vi "FPGA VI_16 Channels_High Speed.vi"() -> ()   [LabVIEW 2015]
uses:
  Types/Injector.Timing.ctl
  Types/Injection.Core.Settings.ctl
  Types/Injection.Global.Settings.ctl
  <vilib>/rvi/eio/common/nirviEmuClasses.ctl
  <vilib>/Platform/TimedLoop/XDataNode/timing_clust.ctl
  <vilib>/Platform/TimedLoop/XDataNode/nitl_modes.ctl
  <vilib>/Platform/TimedLoop/XDataNode/wakeup.ctl
  Types/Injection.Core.Internal.Settings.ctl
  <vilib>/rvi/eio/common/nirviEmuTemplateMethod_errors.vi
  <vilib>/rvi/Emulation/niFpgaGetClockAttributes.vi
  <vilib>/rvi/Emulation/niFpgaSctlEmulationGetInTimedLoop.vi
  <vilib>/rvi/Emulation/niFpgaEmulationReportErrorSimple.vi
  <vilib>/rvi/Emulation/niFpgaCriticalErrorInLSC.vi
  <vilib>/rvi/eio/common/nirviEmuTemplateMethod_noerrors.vi
  <vilib>/rvi/DataTransferAndStorage/Container/Common/niFpgaContainerExecOnDevCompGetState.vi
  <vilib>/rvi/Emulation/niFpgaEmulationIsFPGAContextNoSignature.vi
  <vilib>/rvi/errors/niFpgaSetErrorForExecOnDevCompSimple.vi
  <vilib>/rvi/eio/common/nirviEmuReportErrorAndStop.vi
  <vilib>/rvi/DataTransferAndStorage/Container/Common/niFpgaContainerGetUniqueNameForEmu.vi
  <vilib>/rvi/FIFO/Fifo_Resource/nirvififoEmulationSetSize.vi
  <vilib>/rvi/FIFO/Fifo_Resource/nirviFifoEmulationQueueMgr.vi
  <instcachedir>/0/nirviFifoEmulationQueueMgr_E5CAEC123FF24DC58D834DCA3CDAA9B5.lvgen/nirviFifoEmulationQueueMgr_E5CAEC123FF24DC58D834DCA3CDAA9B5_010.vi
  <vilib>/rvi/FIFO/Fifo_Resource/nirvififoEmulationDetermineInputValidOut.vi
  <vilib>/rvi/FIFO/Fifo_Resource/nirvififoEmulationCreateLock.vi
  <vilib>/rvi/Emulation/niFpgaProcessEmulError.vi
  <vilib>/rvi/FIFO/Fifo_Resource/nirvififoEmulationObtainLock.vi
  <vilib>/rvi/FIFO/Fifo_Resource/nirvififoEmulationReleaseLock.vi
  <vilib>/rvi/occurrence/nirviWaitOnOccurrenceBase.vi
  <vilib>/rvi/errors/nirviReportUnexpectedCaseInternalError.vi
  <vilib>/rvi/errors/nirviReportUnexpectedCaseInternalError (U32).vi
  <vilib>/Utility/error.llb/Clear Errors.vi
  <vilib>/rvi/interface/RandomDataEmulation/niFpgaRandomDataHandleErrors.vi
  <instcachedir>/0/nirviFifoEmulationQueueMgr_E5CAEC123FF24DC58D834DCA3CDAA9B5.lvgen/nirviFifoEmulationQueueMgr_E5CAEC123FF24DC58D834DCA3CDAA9B5_008.vi
  <vilib>/eio/EIOGrowableMethodNode/genericMethod/EIOGrowableMethodNode.xnode
  <vilib>/rvi/eio/nirviEIOMethodImplementation/nirviEIOMethodImplementation.xnode
  <vilib>/rvi/eio/nirviErrorMerge/nirviErrorMerge.xnode
  <vilib>/Platform/TimedLoop/XDataNode/XDataNode.xnode
  <vilib>/rvi/DataTransferAndStorage/Container/XNode/niFpgaContainer.xnode
  <vilib>/rvi/FIFO/Fifo_Resource/niFpgaFifoEmulationRefIn.vi
  <vilib>/rvi/interface/RandomDataEmulation/nirviRandomDataFpgaReadWriteTemplate.vi
  <vilib>/Platform/TimedLoop/XDataNode/XDNodeRunTimeDep.lvlib
panel:
  out "Sample Clock Ticks":u32
  out "Module Error":bool
  out "Module Initialization Error Code":i32
  out "IO Node Timeout":bool
  in  "Settings.Index12.Injector12":T1
  in  "Settings.Index13.Injector13":T1
  in  "Settings.Index14.Injector14":T1
  in  "Settings.Index15.Injector15":T1
  in  "Settings.Index6.Injector6":T1
  in  "Settings.Index7.Injector7":T1
  in  "Settings.Index8.Injector8":T1
  in  "Settings.Index9.Injector9":T1
  in  "Settings.Index10.Injector10":T1
  in  "Settings.Index11.Injector11":T1
  out "Intermediate FIFO Write Timeout":bool
  in  "Settings.Global":T2={"Enable?"=FALSE, "Initial Voltage Threshold"=12.0, "Event Dwell Limit"=2000, "Voltage Gain"=1.0, "Current Gain"=1.0}
  in  "Settings.Index0.Injector0":T1
  in  "Settings.Index1.Injector1":T1
  in  "Settings.Index2.Injector2":T1
  in  "Settings.Index3.Injector3":T1
  in  "Settings.Index4.Injector4":T1
  in  "Settings.Index5.Injector5":T1
  in  "Settings.Timing":T3={"Injector Sample Period (Ticks)"=80}
  out "Acqusition Loop Ticks":u32
  in  "Settings.DMA":cluster{"# of Injectors":u8}={"# of Injectors"=16}
  out "Host DMA Out?":bool
  out "Intermediate Time Out?":bool
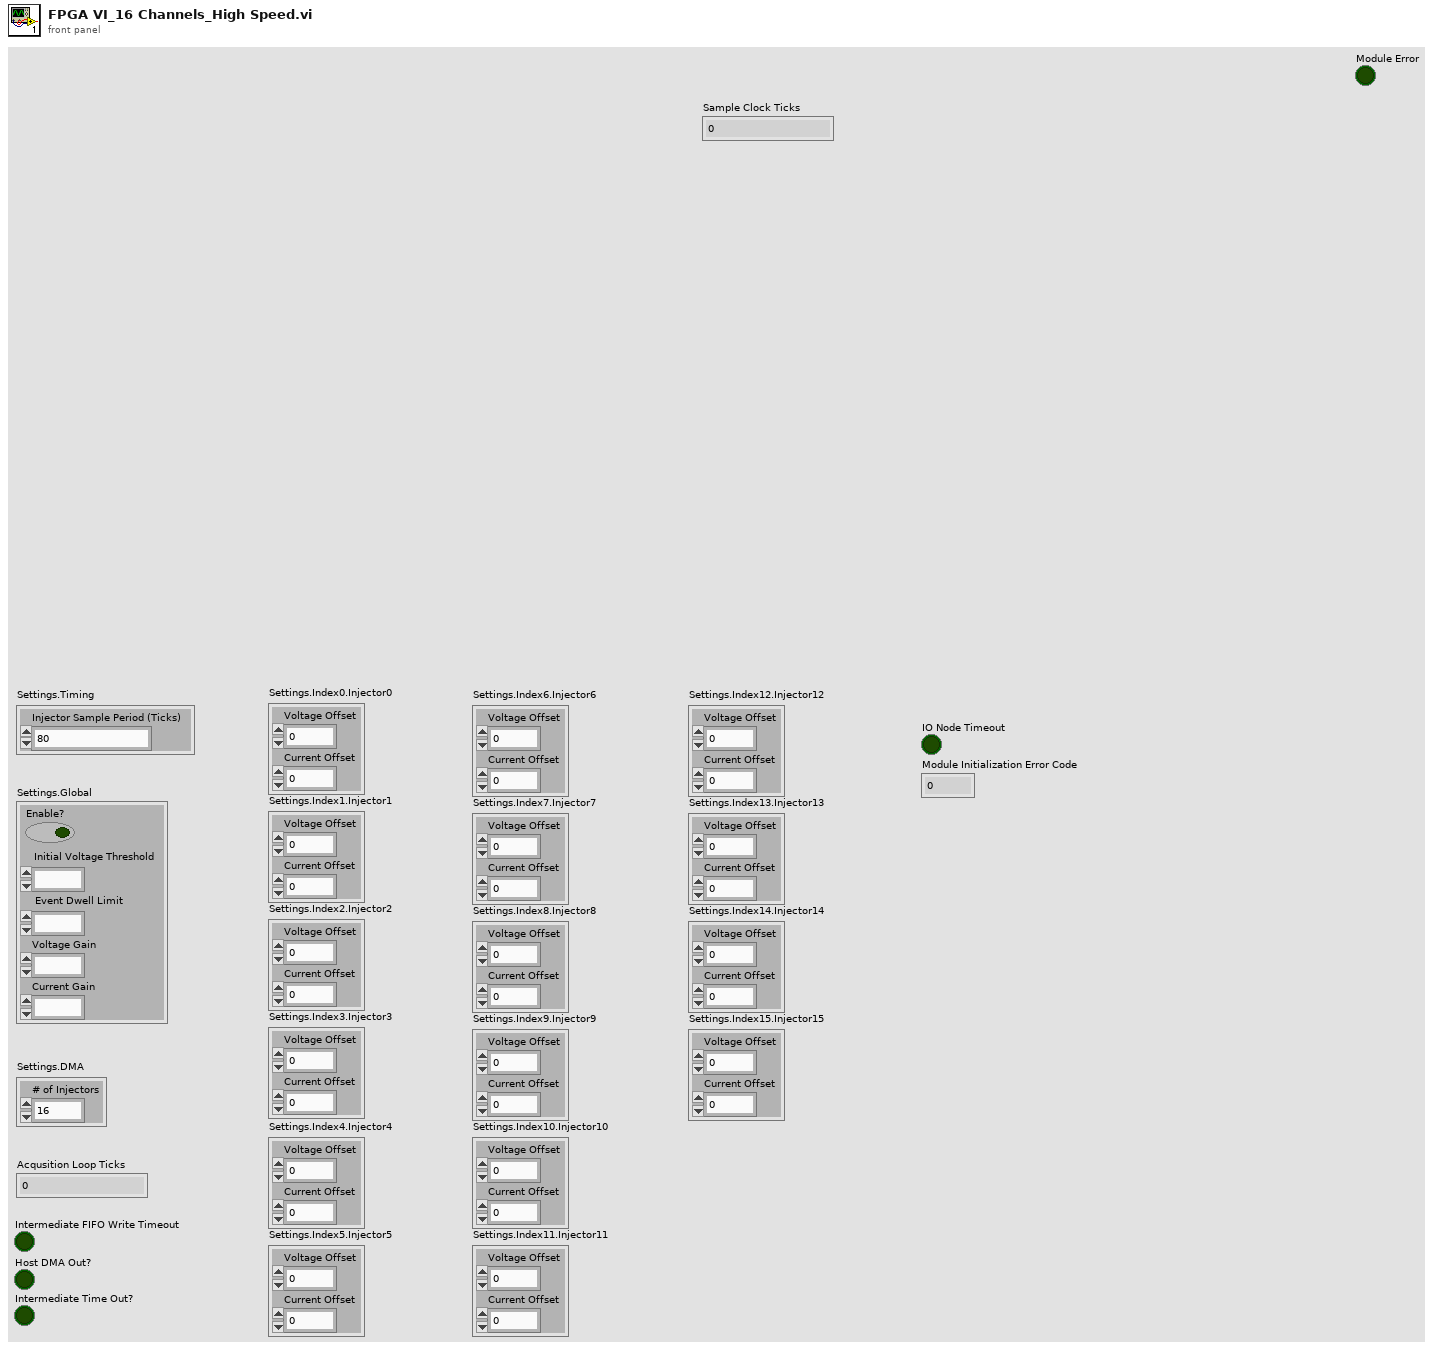
[diagram p1: front panel]
types:
  T1 = typedef "Injection.Core.Settings.ctl" = cluster{"Voltage Offset":fxp<+/-,32,8>, "Current Offset":fxp<+/-,32,8>}
  T2 = typedef "Injection.Global.Settings.ctl" = cluster{"Enable?":bool, "Initial Voltage Threshold":fxp<+/-,32,8>, "Event Dwell Limit":u16, "Voltage Gain":fxp<+/-,32,8>, "Current Gain":fxp<+/-,32,8>}
  T3 = typedef "Injector.Timing.ctl" = cluster{"Injector Sample Period (Ticks)":u32}
  T4 = typedef "nirviEmuClasses.ctl" = enum16{"IO Read", "IO Write", "Method", "Property Read", "Property Write"}
  T5 = cluster{"Data.Samples":u32, "Injection.Period":u32, "Injector.Index":u8, "Iteration":u32}
  T6 = enum8{"Wait on Transfer", "Transfer Injector Index", "Transfer # of Samples", "Transfer Injection Period", "Transfer Data Samples"}
  T7 = typedef "XDNodeRunTimeDep.lvlib/timing_clust.ctl" = cluster{"Expected End [f-1]":u64, "Actual End [f-1]":u64, "Finished Late? [f-1]":bool, "Expected End [i-1]":u64, "Actual End [i-1]":u64, "Finished Late? [i-1]":bool, "Expected Start [i]":u64, "Actual Start [i]":u64, "Expected Start [f]":u64, "Actual Start [f]":u64, "Source Name":string, "Structure Name":string, "Period":i64, "Deadline":i64, "Offset":i64, "Start":i64, "Priority":i32, "Timeout":i32, "Mode":T8, "Wakeup Reason":T9, "Error":errorcluster, "Source Type":string, "Secondary Source Type":string, "Global End Time":u64, "Global Start Time":u64, "Frame Duration":u64, "Iteration Duration":u64, "Assigned CPU":i32, "I/O Scan Engine Mode":u32}
  T8 = typedef "XDNodeRunTimeDep.lvlib/nitl_modes.ctl" = enum32{"No Change", "Process missed periods, maintain original phase", "Discard missed periods, maintain original phase", "Process missed periods, ignore original phase", "Discard missed periods, ignore original phase"}
  T9 = typedef "XDNodeRunTimeDep.lvlib/wakeup.ctl" = enum32{"Normal", "Aborted", "Asynchronous wakeup", "Timing source error", "Timed loop error", "Timeout"}
  T10 = typedef "Injection.Core.Internal.Settings.ctl" = cluster{"Data FIFO":refnum<k21>, "Trigger FIFO":refnum<k21>}
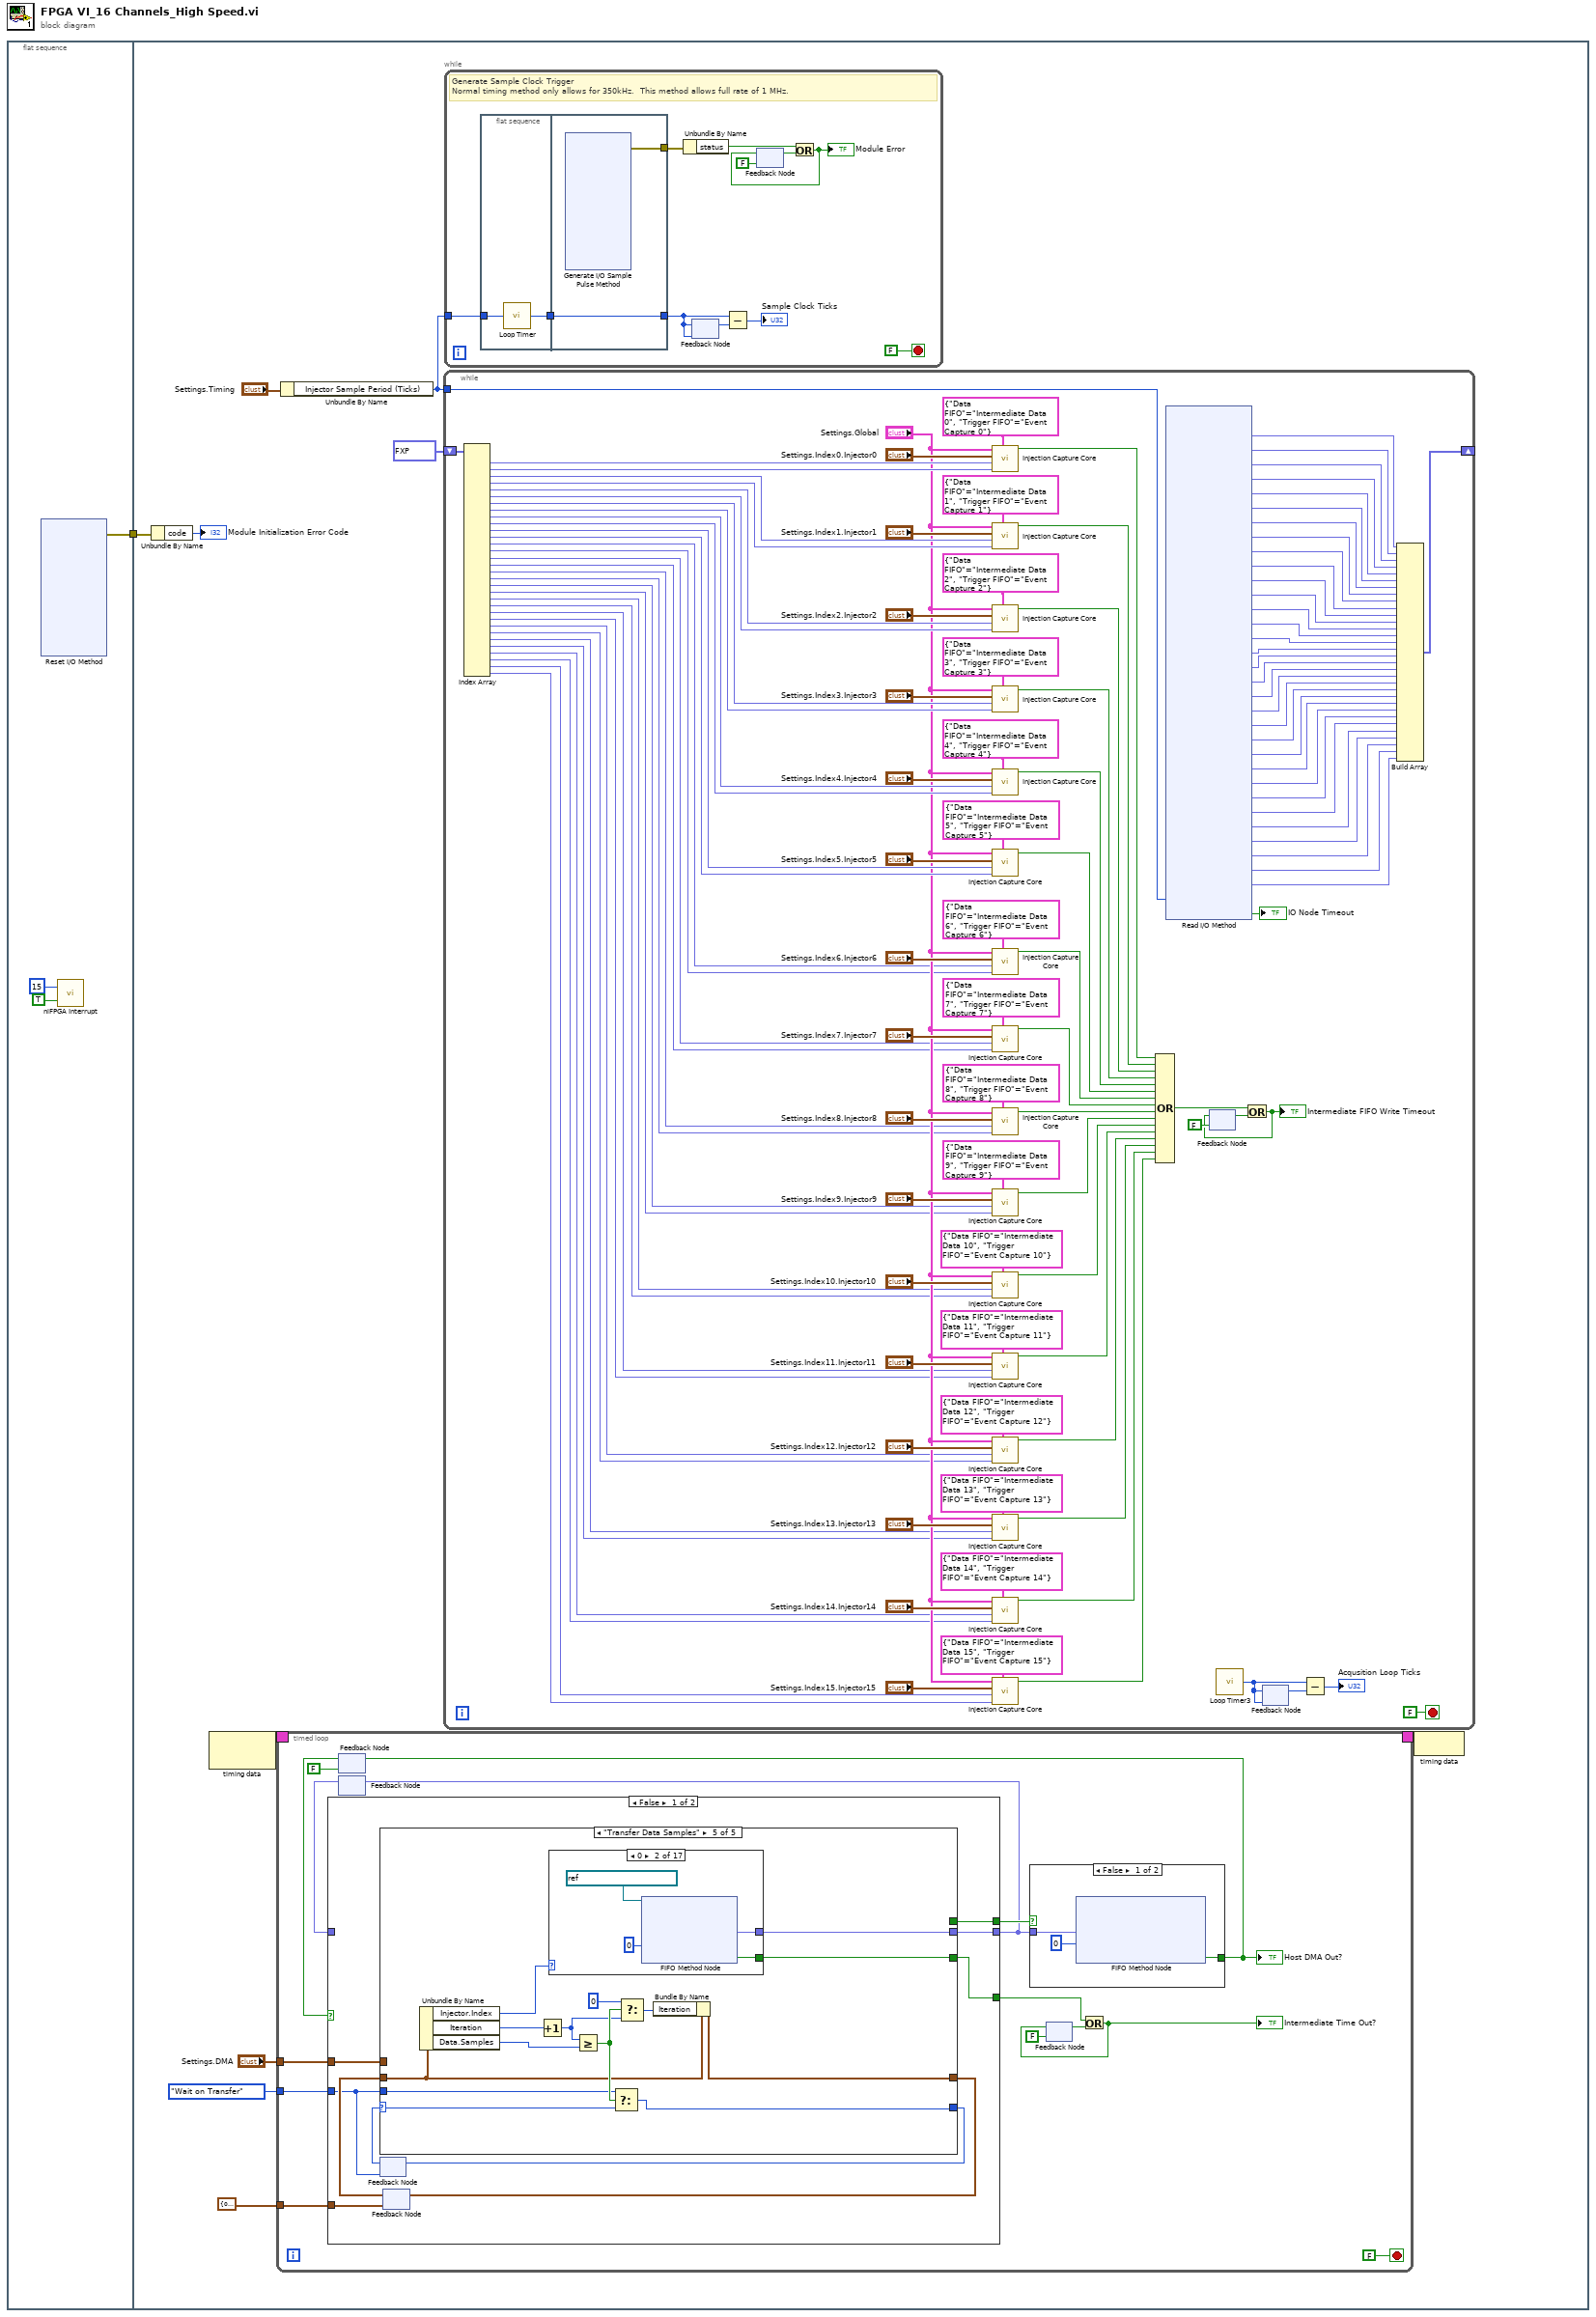
[diagram p0: block diagram]
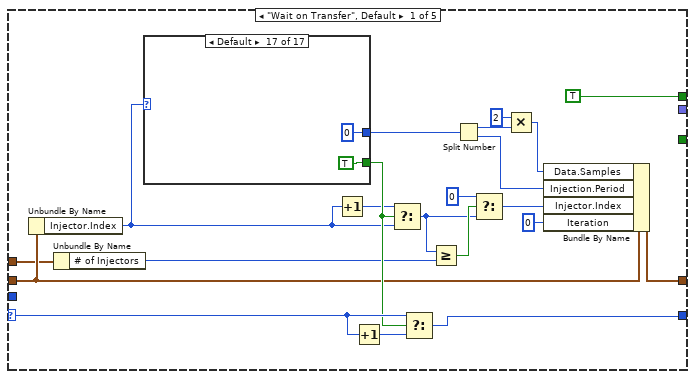
[diagram p2: hidden frame]
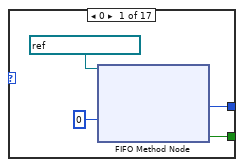
[diagram p3: hidden frame]
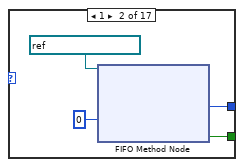
[diagram p4: hidden frame]
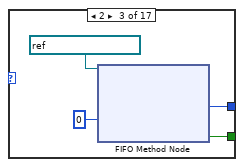
[diagram p5: hidden frame]
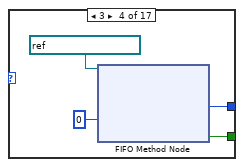
[diagram p6: hidden frame]
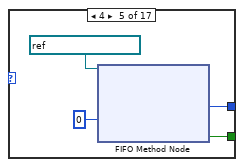
[diagram p7: hidden frame]
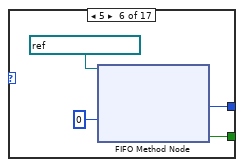
[diagram p8: hidden frame]
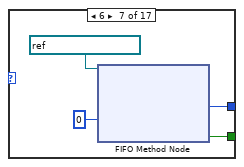
[diagram p9: hidden frame]
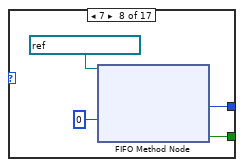
[diagram p10: hidden frame]
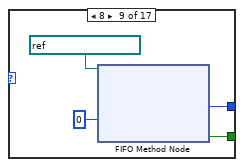
[diagram p11: hidden frame]
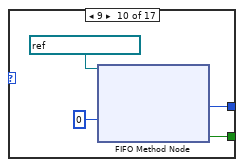
[diagram p12: hidden frame]
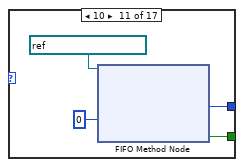
[diagram p13: hidden frame]
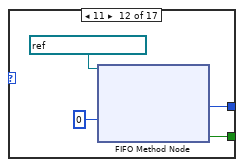
[diagram p14: hidden frame]
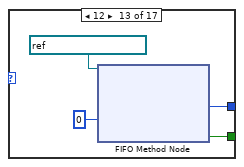
[diagram p15: hidden frame]
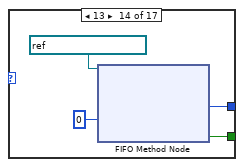
[diagram p16: hidden frame]
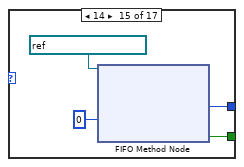
[diagram p17: hidden frame]
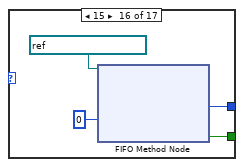
[diagram p18: hidden frame]
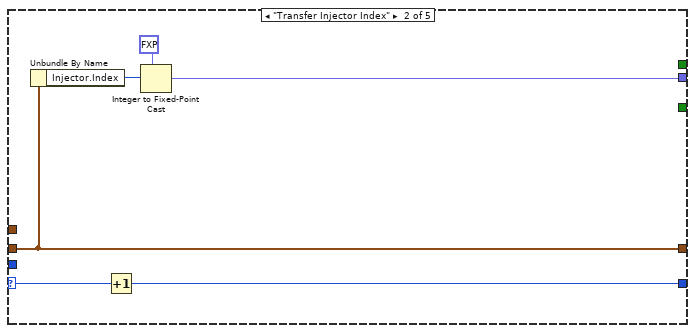
[diagram p19: hidden frame]
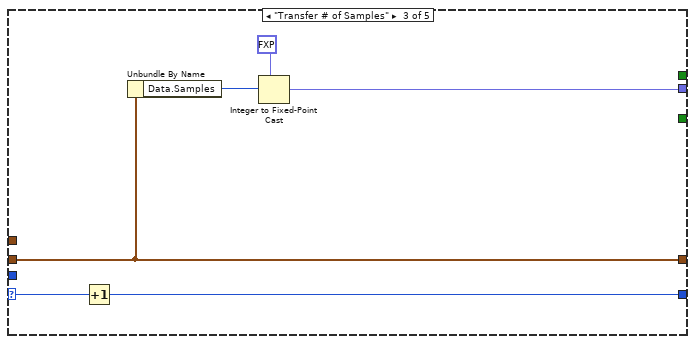
[diagram p20: hidden frame]
diagram:
  n1 = flat-sequence {
    tunnel: [w2] -> w1
    tunnel: w1 -> [w121]
    frame #0 {
      n2 = xnode "Reset I/O Method"() -> ("error out"=w2:errorcluster)  [unwired: 9 in, 8 out]
      n3 = call <vilib>:"niFPGA Interrupt.vi"("Wait Until Cleared (F)"=TRUE, "IRQ Number (0)"=u8 15) -> ()  [unwired: 1 in]
    }
    frame #1 {
      n4 = Unbundle By Name(w121) -> ("code"=→"Module Initialization Error Code":i32)
      n5 = node-c288() -> (w128:T7)  [unwired: 1 in]
      n6 = timed-loop {
        timing: w128 -> [_]
        timing-out: [_] -> w127
        tunnel: "Settings.DMA" -> [w261]
        tunnel: T6."Wait on Transfer" -> [w260]
        tunnel: T5 {"Data.Samples"=0, "Injection.Period"=0, "Injector.Index"=0, "Iteration"=0} ("Local.Data") -> [w259]
        stop <- FALSE stop-if-true
        n7 = feedback #1(FALSE ("Timed Out?")) -> (w269:bool)
        n8 = feedback #2() -> (w266:fxp<+/-,32,8>)  [unwired: 1 in]
        n9 = case shown="False" w269 {
          tunnel: [w281 w466] -> w267
          tunnel: [w280 w465] -> w271
          tunnel: w260 -> [w273 _]
          tunnel: [w278 w465] -> w262
          tunnel: w261 -> [w277 _]
          tunnel: w259 -> [w274 _]
          tunnel: w266 -> [_ w466]
          frame False {
            n10 = feedback #3(w273) -> (w272:T6)
            n11 = feedback #4(w274) -> (w275:T5)
            n12 = case shown="\"Transfer Data Samples\"" w272 {
              selector: w272 -> [w301 w374 w378 w385 w394]
              tunnel: w275 -> [w292 w371 w376 w382 w392]
              tunnel: [w300 w371 w376 w382 w391] -> w276
              tunnel: [w299 w373 w377 w381 w393] -> w279
              tunnel: [_ w370 w375 w384 w390] -> w281
              tunnel: [TRUE _ _ _ _] -> w280
              tunnel: w273 -> [_ _ _ _ w387]
              tunnel: [_ _ _ _ w389] -> w278
              tunnel: w277 -> [w289 _ _ _ _]
              frame "Wait on Transfer", Default {
                n13 = Unbundle By Name(w292) -> ("Injector.Index"=w291:u8)
                n14 = Unbundle By Name(w289) -> ("# of Injectors"=w288:u8)
                n15 = case shown="Default" w291 {
                  tunnel: [w305 w309 w313 w317 w321 w325 w329 w333 w337 w341 w345 w349 w353 w357 w361 w365 u64 0 ("Element")] -> w287
                  tunnel: [w304 w308 w312 w316 w320 w324 w328 w332 w336 w340 w344 w348 w352 w356 w360 w364 TRUE ("Timed Out?")] -> w297
                  frame 0 {
                    n16 = xnode ("FIFO Method Node")("Timeout"=0, "FIFO In"=refnum<k21> "Event Capture 0") -> ("Element"=w305:u64, "Timed Out?"=w304:bool)  [unwired: 1 out]
                  }
                  frame 1 {
                    n17 = xnode ("FIFO Method Node")("Timeout"=0, "FIFO In"=refnum<k21> "Event Capture 1") -> ("Element"=w309:u64, "Timed Out?"=w308:bool)  [unwired: 1 out]
                  }
                  frame 2 {
                    n18 = xnode ("FIFO Method Node")("Timeout"=0, "FIFO In"=refnum<k21> "Event Capture 2") -> ("Element"=w313:u64, "Timed Out?"=w312:bool)  [unwired: 1 out]
                  }
                  frame 3 {
                    n19 = xnode ("FIFO Method Node")("Timeout"=0, "FIFO In"=refnum<k21> "Event Capture 3") -> ("Element"=w317:u64, "Timed Out?"=w316:bool)  [unwired: 1 out]
                  }
                  frame 4 {
                    n20 = xnode ("FIFO Method Node")("Timeout"=0, "FIFO In"=refnum<k21> "Event Capture 4") -> ("Element"=w321:u64, "Timed Out?"=w320:bool)  [unwired: 1 out]
                  }
                  frame 5 {
                    n21 = xnode ("FIFO Method Node")("Timeout"=0, "FIFO In"=refnum<k21> "Event Capture 5") -> ("Element"=w325:u64, "Timed Out?"=w324:bool)  [unwired: 1 out]
                  }
                  frame 6 {
                    n22 = xnode ("FIFO Method Node")("Timeout"=0, "FIFO In"=refnum<k21> "Event Capture 6") -> ("Element"=w329:u64, "Timed Out?"=w328:bool)  [unwired: 1 out]
                  }
                  frame 7 {
                    n23 = xnode ("FIFO Method Node")("Timeout"=0, "FIFO In"=refnum<k21> "Event Capture 7") -> ("Element"=w333:u64, "Timed Out?"=w332:bool)  [unwired: 1 out]
                  }
                  frame 8 {
                    n24 = xnode ("FIFO Method Node")("Timeout"=0, "FIFO In"=refnum<k21> "Event Capture 8") -> ("Element"=w337:u64, "Timed Out?"=w336:bool)  [unwired: 1 out]
                  }
                  frame 9 {
                    n25 = xnode ("FIFO Method Node")("Timeout"=0, "FIFO In"=refnum<k21> "Event Capture 9") -> ("Element"=w341:u64, "Timed Out?"=w340:bool)  [unwired: 1 out]
                  }
                  frame 10 {
                    n26 = xnode ("FIFO Method Node")("Timeout"=0, "FIFO In"=refnum<k21> "Event Capture 10") -> ("Element"=w345:u64, "Timed Out?"=w344:bool)  [unwired: 1 out]
                  }
                  frame 11 {
                    n27 = xnode ("FIFO Method Node")("Timeout"=0, "FIFO In"=refnum<k21> "Event Capture 11") -> ("Element"=w349:u64, "Timed Out?"=w348:bool)  [unwired: 1 out]
                  }
                  frame 12 {
                    n28 = xnode ("FIFO Method Node")("Timeout"=0, "FIFO In"=refnum<k21> "Event Capture 12") -> ("Element"=w353:u64, "Timed Out?"=w352:bool)  [unwired: 1 out]
                  }
                  frame 13 {
                    n29 = xnode ("FIFO Method Node")("Timeout"=0, "FIFO In"=refnum<k21> "Event Capture 13") -> ("Element"=w357:u64, "Timed Out?"=w356:bool)  [unwired: 1 out]
                  }
                  frame 14 {
                    n30 = xnode ("FIFO Method Node")("Timeout"=0, "FIFO In"=refnum<k21> "Event Capture 14") -> ("Element"=w361:u64, "Timed Out?"=w360:bool)  [unwired: 1 out]
                  }
                  frame 15 {
                    n31 = xnode ("FIFO Method Node")("Timeout"=0, "FIFO In"=refnum<k21> "Event Capture 15") -> ("Element"=w365:u64, "Timed Out?"=w364:bool)  [unwired: 1 out]
                  }
                  frame Default {
                  }
                }
                n32 = Increment(x=w291) -> (x+1=w296:u8)
                n33 = Increment(x=w301) -> (x+1=w302:T6)
                n34 = Select(t=w296, s=w297, f=w291) -> (s? t:f=w294:u8)
                n35 = Select(t=w301, s=w297, f=w302) -> (s? t:f=w299:T6)
                n36 = Greater Or Equal?(x=w294, y=w288) -> (x >= y?=w295:bool)
                n37 = Split Number(x=w287) -> (hi(x)=w286:u32, lo(x)=w285:u32)
                n38 = Select(t=u8 0, s=w295, f=w294) -> (s? t:f=w290:u8)
                n39 = Multiply(x=u32 2, y=w286) -> (x*y=w283:u32)
                n40 = Bundle By Name(cluster=w292, "Data.Samples"=w283, "Injection.Period"=w285, "Injector.Index"=w290, "Iteration"=u32 0) -> (w300:T5)
              }
              frame "Transfer Injector Index" {
                n41 = Unbundle By Name(w371) -> ("Injector.Index"=w372:u8)
                n42 = Increment(x=w374) -> (x+1=w373:T6)
                n43 = Integer to Fixed-Point Cast(fixed-point type=fxp<+/-,32,8> 0.0, integer=w372) -> (fixed-point=w370:fxp<+/-,32,8>)
              }
              frame "Transfer # of Samples" {
                n44 = Increment(x=w378) -> (x+1=w377:T6)
                n45 = Unbundle By Name(w376) -> ("Data.Samples"=w379:u32)
                n46 = Integer to Fixed-Point Cast(fixed-point type=fxp<+/-,32,8> 0.0, integer=w379) -> (fixed-point=w375:fxp<+/-,32,8>)
              }
              frame "Transfer Injection Period" {
                n47 = Unbundle By Name(w382) -> ("Injection.Period"=w383:u32)
                n48 = Increment(x=w385) -> (x+1=w381:T6)
                n49 = Integer to Fixed-Point Cast(fixed-point type=fxp<+/-,32,8> 0.0, integer=w383) -> (fixed-point=w384:fxp<+/-,32,8>)
              }
              frame "Transfer Data Samples" {
                n50 = Unbundle By Name(w392) -> ("Injector.Index"=w400:u8, "Iteration"=w395:u32, "Data.Samples"=w388:u32)
                n51 = Increment(x=w395) -> (x+1=w397:u32)
                n52 = case shown="0" w400 {
                  tunnel: [_ w403 w407 w411 w415 w419 w423 w427 w431 w435 w439 w443 w447 w451 w455 w459 w463] -> w390
                  tunnel: [_ w402 w406 w410 w414 w418 w422 w426 w430 w434 w438 w442 w446 w450 w454 w458 w462] -> w389
                  frame Default {
                  }
                  frame 0 {
                    n53 = xnode ("FIFO Method Node")("Timeout"=0, "FIFO In"=refnum<k21> "Intermediate Data 0" ("Voltage FIFO")) -> ("Element"=w403:fxp<+/-,32,8>, "Timed Out?"=w402:bool)  [unwired: 1 out]
                  }
                  frame 1 {
                    n54 = xnode ("FIFO Method Node")("Timeout"=0, "FIFO In"=refnum<k21> "Intermediate Data 1" ("Voltage FIFO")) -> ("Element"=w407:fxp<+/-,32,8>, "Timed Out?"=w406:bool)  [unwired: 1 out]
                  }
                  frame 2 {
                    n55 = xnode ("FIFO Method Node")("Timeout"=0, "FIFO In"=refnum<k21> "Intermediate Data 2" ("Voltage FIFO")) -> ("Element"=w411:fxp<+/-,32,8>, "Timed Out?"=w410:bool)  [unwired: 1 out]
                  }
                  frame 3 {
                    n56 = xnode ("FIFO Method Node")("Timeout"=0, "FIFO In"=refnum<k21> "Intermediate Data 3" ("Voltage FIFO")) -> ("Element"=w415:fxp<+/-,32,8>, "Timed Out?"=w414:bool)  [unwired: 1 out]
                  }
                  frame 4 {
                    n57 = xnode ("FIFO Method Node")("Timeout"=0, "FIFO In"=refnum<k21> "Intermediate Data 4" ("Voltage FIFO")) -> ("Element"=w419:fxp<+/-,32,8>, "Timed Out?"=w418:bool)  [unwired: 1 out]
                  }
                  frame 5 {
                    n58 = xnode ("FIFO Method Node")("Timeout"=0, "FIFO In"=refnum<k21> "Intermediate Data 5" ("Voltage FIFO")) -> ("Element"=w423:fxp<+/-,32,8>, "Timed Out?"=w422:bool)  [unwired: 1 out]
                  }
                  frame 6 {
                    n59 = xnode ("FIFO Method Node")("Timeout"=0, "FIFO In"=refnum<k21> "Intermediate Data 6" ("Voltage FIFO")) -> ("Element"=w427:fxp<+/-,32,8>, "Timed Out?"=w426:bool)  [unwired: 1 out]
                  }
                  frame 7 {
                    n60 = xnode ("FIFO Method Node")("Timeout"=0, "FIFO In"=refnum<k21> "Intermediate Data 7" ("Voltage FIFO")) -> ("Element"=w431:fxp<+/-,32,8>, "Timed Out?"=w430:bool)  [unwired: 1 out]
                  }
                  frame 8 {
                    n61 = xnode ("FIFO Method Node")("Timeout"=0, "FIFO In"=refnum<k21> "Intermediate Data 8" ("Voltage FIFO")) -> ("Element"=w435:fxp<+/-,32,8>, "Timed Out?"=w434:bool)  [unwired: 1 out]
                  }
                  frame 9 {
                    n62 = xnode ("FIFO Method Node")("Timeout"=0, "FIFO In"=refnum<k21> "Intermediate Data 9" ("Voltage FIFO")) -> ("Element"=w439:fxp<+/-,32,8>, "Timed Out?"=w438:bool)  [unwired: 1 out]
                  }
                  frame 10 {
                    n63 = xnode ("FIFO Method Node")("Timeout"=0, "FIFO In"=refnum<k21> "Intermediate Data 10" ("Voltage FIFO")) -> ("Element"=w443:fxp<+/-,32,8>, "Timed Out?"=w442:bool)  [unwired: 1 out]
                  }
                  frame 11 {
                    n64 = xnode ("FIFO Method Node")("Timeout"=0, "FIFO In"=refnum<k21> "Intermediate Data 11" ("Voltage FIFO")) -> ("Element"=w447:fxp<+/-,32,8>, "Timed Out?"=w446:bool)  [unwired: 1 out]
                  }
                  frame 12 {
                    n65 = xnode ("FIFO Method Node")("Timeout"=0, "FIFO In"=refnum<k21> "Intermediate Data 12" ("Voltage FIFO")) -> ("Element"=w451:fxp<+/-,32,8>, "Timed Out?"=w450:bool)  [unwired: 1 out]
                  }
                  frame 13 {
                    n66 = xnode ("FIFO Method Node")("Timeout"=0, "FIFO In"=refnum<k21> "Intermediate Data 13" ("Voltage FIFO")) -> ("Element"=w455:fxp<+/-,32,8>, "Timed Out?"=w454:bool)  [unwired: 1 out]
                  }
                  frame 14 {
                    n67 = xnode ("FIFO Method Node")("Timeout"=0, "FIFO In"=refnum<k21> "Intermediate Data 14" ("Voltage FIFO")) -> ("Element"=w459:fxp<+/-,32,8>, "Timed Out?"=w458:bool)  [unwired: 1 out]
                  }
                  frame 15 {
                    n68 = xnode ("FIFO Method Node")("Timeout"=0, "FIFO In"=refnum<k21> "Intermediate Data 15" ("Voltage FIFO")) -> ("Element"=w463:fxp<+/-,32,8>, "Timed Out?"=w462:bool)  [unwired: 1 out]
                  }
                }
                n69 = Greater Or Equal?(x=w397, y=w388) -> (x >= y?=w399:bool)
                n70 = Select(t=w387, s=w399, f=w394) -> (s? t:f=w393:T6)
                n71 = Select(t=u32 0, s=w399, f=w397) -> (s? t:f=w396:u32)
                n72 = Bundle By Name(cluster=w392, "Iteration"=w396) -> (w391:T5)
              }
            }
            n73 = feedback-in #3(w279) -> ()
            n74 = feedback-in #4(w276) -> ()
          }
          frame True {
            w465 = FALSE
          }
        }
        n75 = feedback-in #2(w267) -> ()
        n76 = case shown="False" w271 {
          tunnel: w267 -> [w468 _]
          tunnel: [w467 FALSE ("Timed Out?")] -> w270
          frame False {
            n77 = xnode ("FIFO Method Node")("Element"=w468, "Timeout"=0) -> ("Timed Out?"=w467:bool)  [unwired: 1 in, 1 out]
          }
          frame True {
          }
        }
        "Host DMA Out?" <- w270
        n78 = feedback-in #1(w270) -> ()
        n79 = feedback #5(FALSE ("Timed Out?")) -> (w264:bool)
        n80 = Or(x=w262, y=w264) -> (x .or. y?=w263:bool)
        "Intermediate Time Out?" <- w263
        n81 = feedback-in #5(w263) -> ()
      }
      n82 = Unbundle By Name("Settings.Timing") -> ("Injector Sample Period (Ticks)"=w119:u32)
      n83 = while {
        shift-right: [w560] -> _
        shift-left: fxp<+/-,24,5>[] [0.0, 0.0, 0.0, 0.0, 0.0, 0.0, 0.0, 0.0, 0.0, 0.0, 0.0, 0.0, 0.0, 0.0, 0.0, 0.0, 0.0, 0.0, 0.0, 0.0, 0.0, 0.0, 0.0, 0.0, 0.0, 0.0, 0.0, 0.0, 0.0, 0.0, 0.0, 0.0] -> [w580]
        tunnel: w119 -> [w475]
        stop <- FALSE stop-if-true
        n84 = Index Array(array=w580) -> (element #1=w591:fxp<+/-,24,5>, element #2=w592:fxp<+/-,24,5>, element #3=w589:fxp<+/-,24,5>, element #4=w590:fxp<+/-,24,5>, element #5=w587:fxp<+/-,24,5>, element #6=w588:fxp<+/-,24,5>, element #7=w585:fxp<+/-,24,5>, element #8=w586:fxp<+/-,24,5>, element #9=w583:fxp<+/-,24,5>, element #10=w584:fxp<+/-,24,5>, element #11=w581:fxp<+/-,24,5>, element #12=w582:fxp<+/-,24,5>, element #13=w528:fxp<+/-,24,5>, element #14=w527:fxp<+/-,24,5>, element #15=w526:fxp<+/-,24,5>, element #16=w525:fxp<+/-,24,5>, element #17=w524:fxp<+/-,24,5>, element #18=w523:fxp<+/-,24,5>, element #19=w522:fxp<+/-,24,5>, element #20=w521:fxp<+/-,24,5>, element #21=w520:fxp<+/-,24,5>, element #22=w519:fxp<+/-,24,5>, element #23=w518:fxp<+/-,24,5>, element #24=w517:fxp<+/-,24,5>, element #25=w516:fxp<+/-,24,5>, element #26=w515:fxp<+/-,24,5>, element #27=w514:fxp<+/-,24,5>, element #28=w513:fxp<+/-,24,5>, element #29=w512:fxp<+/-,24,5>, element #30=w511:fxp<+/-,24,5>, element #31=w510:fxp<+/-,24,5>, element #32=w509:fxp<+/-,24,5>)  [unwired: 32 in]
        n85 = call "Injection Capture Core.vi"("FIFOs"=T10 {"Data FIFO"="Intermediate Data 0", "Trigger FIFO"="Event Capture 0"} ("InjectorCore.Settings"), "Current (PreScaled)"=w592, "Voltage (PreScaled)"=w591, "Settings.Index<#>.<UserName>"="Settings.Index0.Injector0", "Settings.Global"="Settings.Global") -> ("Intermediate FIFO Timeout?"=w599:bool)  [unwired: 4 in, 2 out]
        n86 = call "Injection Capture Core.vi"("FIFOs"=T10 {"Data FIFO"="Intermediate Data 1", "Trigger FIFO"="Event Capture 1"} ("InjectorCore.Settings"), "Current (PreScaled)"=w590, "Voltage (PreScaled)"=w589, "Settings.Index<#>.<UserName>"="Settings.Index1.Injector1", "Settings.Global"="Settings.Global") -> ("Intermediate FIFO Timeout?"=w598:bool)  [unwired: 4 in, 2 out]
        n87 = call "Injection Capture Core.vi"("FIFOs"=T10 {"Data FIFO"="Intermediate Data 2", "Trigger FIFO"="Event Capture 2"} ("InjectorCore.Settings"), "Current (PreScaled)"=w588, "Voltage (PreScaled)"=w587, "Settings.Index<#>.<UserName>"="Settings.Index2.Injector2", "Settings.Global"="Settings.Global") -> ("Intermediate FIFO Timeout?"=w597:bool)  [unwired: 4 in, 2 out]
        n88 = call "Injection Capture Core.vi"("FIFOs"=T10 {"Data FIFO"="Intermediate Data 3", "Trigger FIFO"="Event Capture 3"} ("InjectorCore.Settings"), "Current (PreScaled)"=w586, "Voltage (PreScaled)"=w585, "Settings.Index<#>.<UserName>"="Settings.Index3.Injector3", "Settings.Global"="Settings.Global") -> ("Intermediate FIFO Timeout?"=w596:bool)  [unwired: 4 in, 2 out]
        n89 = call "Injection Capture Core.vi"("FIFOs"=T10 {"Data FIFO"="Intermediate Data 4", "Trigger FIFO"="Event Capture 4"} ("InjectorCore.Settings"), "Current (PreScaled)"=w584, "Voltage (PreScaled)"=w583, "Settings.Index<#>.<UserName>"="Settings.Index4.Injector4", "Settings.Global"="Settings.Global") -> ("Intermediate FIFO Timeout?"=w595:bool)  [unwired: 4 in, 2 out]
        n90 = call "Injection Capture Core.vi"("FIFOs"=T10 {"Data FIFO"="Intermediate Data 5", "Trigger FIFO"="Event Capture 5"} ("InjectorCore.Settings"), "Current (PreScaled)"=w582, "Voltage (PreScaled)"=w581, "Settings.Index<#>.<UserName>"="Settings.Index5.Injector5", "Settings.Global"="Settings.Global") -> ("Intermediate FIFO Timeout?"=w594:bool)  [unwired: 4 in, 2 out]
        n91 = call "Injection Capture Core.vi"("FIFOs"=T10 {"Data FIFO"="Intermediate Data 6", "Trigger FIFO"="Event Capture 6"} ("InjectorCore.Settings"), "Current (PreScaled)"=w527, "Voltage (PreScaled)"=w528, "Settings.Index<#>.<UserName>"="Settings.Index6.Injector6", "Settings.Global"="Settings.Global") -> ("Intermediate FIFO Timeout?"=w538:bool)  [unwired: 4 in, 2 out]
        n92 = call "Injection Capture Core.vi"("FIFOs"=T10 {"Data FIFO"="Intermediate Data 7", "Trigger FIFO"="Event Capture 7"} ("InjectorCore.Settings"), "Current (PreScaled)"=w525, "Voltage (PreScaled)"=w526, "Settings.Index<#>.<UserName>"="Settings.Index7.Injector7", "Settings.Global"="Settings.Global") -> ("Intermediate FIFO Timeout?"=w537:bool)  [unwired: 4 in, 2 out]
        n93 = call "Injection Capture Core.vi"("FIFOs"=T10 {"Data FIFO"="Intermediate Data 8", "Trigger FIFO"="Event Capture 8"} ("InjectorCore.Settings"), "Current (PreScaled)"=w523, "Voltage (PreScaled)"=w524, "Settings.Index<#>.<UserName>"="Settings.Index8.Injector8", "Settings.Global"="Settings.Global") -> ("Intermediate FIFO Timeout?"=w536:bool)  [unwired: 4 in, 2 out]
        n94 = call "Injection Capture Core.vi"("FIFOs"=T10 {"Data FIFO"="Intermediate Data 9", "Trigger FIFO"="Event Capture 9"} ("InjectorCore.Settings"), "Current (PreScaled)"=w521, "Voltage (PreScaled)"=w522, "Settings.Index<#>.<UserName>"="Settings.Index9.Injector9", "Settings.Global"="Settings.Global") -> ("Intermediate FIFO Timeout?"=w535:bool)  [unwired: 4 in, 2 out]
        n95 = call "Injection Capture Core.vi"("FIFOs"=T10 {"Data FIFO"="Intermediate Data 10", "Trigger FIFO"="Event Capture 10"} ("InjectorCore.Settings"), "Current (PreScaled)"=w519, "Voltage (PreScaled)"=w520, "Settings.Index<#>.<UserName>"="Settings.Index10.Injector10", "Settings.Global"="Settings.Global") -> ("Intermediate FIFO Timeout?"=w534:bool)  [unwired: 4 in, 2 out]
        n96 = call "Injection Capture Core.vi"("FIFOs"=T10 {"Data FIFO"="Intermediate Data 11", "Trigger FIFO"="Event Capture 11"} ("InjectorCore.Settings"), "Current (PreScaled)"=w517, "Voltage (PreScaled)"=w518, "Settings.Index<#>.<UserName>"="Settings.Index11.Injector11", "Settings.Global"="Settings.Global") -> ("Intermediate FIFO Timeout?"=w533:bool)  [unwired: 4 in, 2 out]
        n97 = call "Injection Capture Core.vi"("FIFOs"=T10 {"Data FIFO"="Intermediate Data 12", "Trigger FIFO"="Event Capture 12"} ("InjectorCore.Settings"), "Current (PreScaled)"=w515, "Voltage (PreScaled)"=w516, "Settings.Index<#>.<UserName>"="Settings.Index12.Injector12", "Settings.Global"="Settings.Global") -> ("Intermediate FIFO Timeout?"=w532:bool)  [unwired: 4 in, 2 out]
        n98 = call "Injection Capture Core.vi"("FIFOs"=T10 {"Data FIFO"="Intermediate Data 13", "Trigger FIFO"="Event Capture 13"} ("InjectorCore.Settings"), "Current (PreScaled)"=w513, "Voltage (PreScaled)"=w514, "Settings.Index<#>.<UserName>"="Settings.Index13.Injector13", "Settings.Global"="Settings.Global") -> ("Intermediate FIFO Timeout?"=w531:bool)  [unwired: 4 in, 2 out]
        n99 = call "Injection Capture Core.vi"("FIFOs"=T10 {"Data FIFO"="Intermediate Data 14", "Trigger FIFO"="Event Capture 14"} ("InjectorCore.Settings"), "Current (PreScaled)"=w511, "Voltage (PreScaled)"=w512, "Settings.Index<#>.<UserName>"="Settings.Index14.Injector14", "Settings.Global"="Settings.Global") -> ("Intermediate FIFO Timeout?"=w530:bool)  [unwired: 4 in, 2 out]
        n100 = call "Injection Capture Core.vi"("FIFOs"=T10 {"Data FIFO"="Intermediate Data 15", "Trigger FIFO"="Event Capture 15"} ("InjectorCore.Settings"), "Current (PreScaled)"=w509, "Voltage (PreScaled)"=w510, "Settings.Index<#>.<UserName>"="Settings.Index15.Injector15", "Settings.Global"="Settings.Global") -> ("Intermediate FIFO Timeout?"=w529:bool)  [unwired: 4 in, 2 out]
        n101 = Compound Arithmetic op=OR(w599, w598, w597, w596, w595, w594, w538, w537, w536, w535, w534, w533, w532, w531, w530, w529) -> (w570:bool)
        n102 = xnode "Read I/O Method"("Timeout"=w475) -> ("Mod1/AI0"=w508:fxp<+/-,24,5>, "Mod1/AI1"=w507:fxp<+/-,24,5>, "Mod1/AI2"=w506:fxp<+/-,24,5>, "Mod1/AI3"=w505:fxp<+/-,24,5>, "Mod2/AI0"=w504:fxp<+/-,24,5>, "Mod2/AI1"=w503:fxp<+/-,24,5>, "Mod2/AI2"=w502:fxp<+/-,24,5>, "Mod2/AI3"=w501:fxp<+/-,24,5>, "Mod3/AI0"=w500:fxp<+/-,24,5>, "Mod3/AI1"=w499:fxp<+/-,24,5>, "Mod3/AI2"=w498:fxp<+/-,24,5>, "Mod3/AI3"=w497:fxp<+/-,24,5>, "Mod4/AI0"=w496:fxp<+/-,24,5>, "Mod4/AI1"=w495:fxp<+/-,24,5>, "Mod4/AI2"=w494:fxp<+/-,24,5>, "Mod4/AI3"=w493:fxp<+/-,24,5>, "Mod5/AI0"=w492:fxp<+/-,24,5>, "Mod5/AI1"=w491:fxp<+/-,24,5>, "Mod5/AI2"=w490:fxp<+/-,24,5>, "Mod5/AI3"=w489:fxp<+/-,24,5>, "Mod6/AI0"=w488:fxp<+/-,24,5>, "Mod6/AI1"=w487:fxp<+/-,24,5>, "Mod6/AI2"=w486:fxp<+/-,24,5>, "Mod6/AI3"=w485:fxp<+/-,24,5>, "Mod7/AI0"=w484:fxp<+/-,24,5>, "Mod7/AI1"=w483:fxp<+/-,24,5>, "Mod7/AI2"=w482:fxp<+/-,24,5>, "Mod7/AI3"=w481:fxp<+/-,24,5>, "Mod8/AI0"=w480:fxp<+/-,24,5>, "Mod8/AI1"=w479:fxp<+/-,24,5>, "Mod8/AI2"=w478:fxp<+/-,24,5>, "Mod8/AI3"=w477:fxp<+/-,24,5>, "Timed Out"=→"IO Node Timeout":bool)  [unwired: 33 in, 33 out]
        n103 = feedback #6(FALSE ("Timed Out?")) -> (w571:bool)
        n104 = call "Loop Timer3"() -> ("Tick Count(Ticks)"=w566:u32)  [unwired: 1 in]
        n105 = Or(x=w570, y=w571) -> (x .or. y?=w569:bool)
        "Intermediate FIFO Write Timeout" <- w569
        n106 = feedback-in #6(w569) -> ()
        n107 = feedback-in #7(w566) -> ()
        n108 = feedback #7(w566) -> (w568:u32)
        n109 = Subtract(x=w566, y=w568) -> (x-y=→"Acqusition Loop Ticks":u32)
        n110 = Build Array(w508, w507, w506, w505, w504, w503, w502, w501, w500, w499, w498, w497, w496, w495, w494, w493, w492, w491, w490, w489, w488, w487, w486, w485, w484, w483, w482, w481, w480, w479, w478, w477) -> (w560:fxp<+/-,24,5>[])
      }
      n111 = while {
        tunnel: w119 -> [w138]
        stop <- FALSE stop-if-true
        # "Generate Sample Clock Trigger\nNormal timing method only allows for 350kHz.  This method allows full rate of 1 MHz."
        n112 = flat-sequence {
          tunnel: w138 -> [w141]
          tunnel: [w140] -> w129
          tunnel: [w143] -> w139
          tunnel: [w142] -> w130
          tunnel: w129 -> [w142]
          frame #0 {
            n113 = call "Loop Timer"("Count(Ticks)"=w141) -> ("Tick Count(Ticks)"=w140:u32)
          }
          frame #1 {
            n114 = xnode "Generate I/O Sample Pulse Method"() -> ("error out"=w143:errorcluster)  [unwired: 9 in, 8 out]
          }
        }
        n115 = Unbundle By Name(w139) -> ("status"=w131:bool)
        n116 = feedback #8(w130) -> (w136:u32)
        n117 = feedback-in #8(w130) -> ()
        n118 = Subtract(x=w130, y=w136) -> (x-y=→"Sample Clock Ticks":u32)
        n119 = feedback #9(FALSE ("Timed Out?")) -> (w133:bool)
        n120 = Or(x=w131, y=w133) -> (x .or. y?=w132:bool)
        "Module Error" <- w132
        n121 = feedback-in #9(w132) -> ()
      }
      n122 = node-c288(w127) -> ()
    }
  }
